vi "TEST - Wait Until Next ms Multiple.vi"(8 "error in (no error)":errorcluster) -> (0 "error out":errorcluster, 2 "pass":bool)   [LabVIEW 2020]
uses:
  source/library/openg_time.lvlib
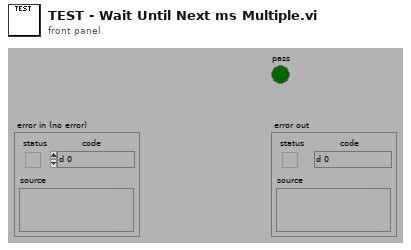
[diagram p1: front panel]
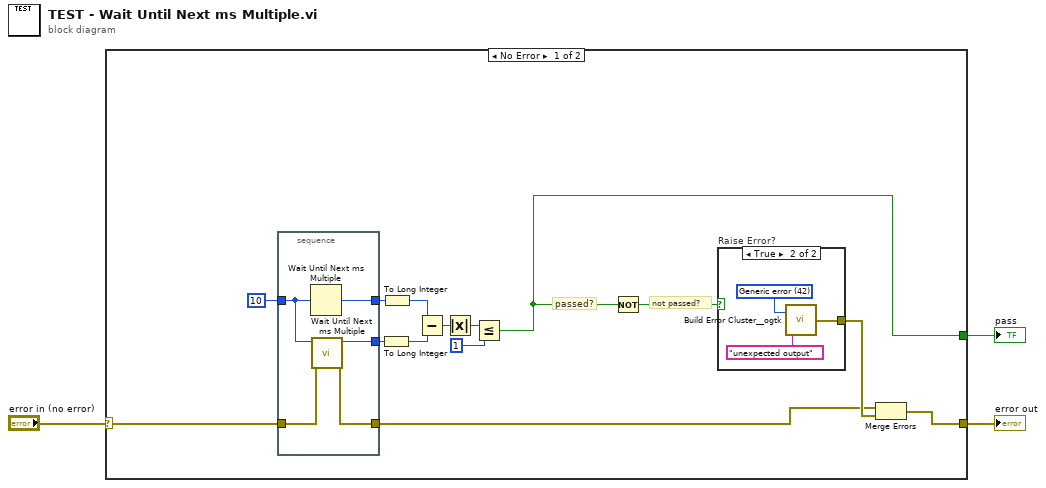
[diagram p0: block diagram]
diagram:
  n1 = case shown="No Error" "error in (no error)" {
    selector: "error in (no error)" -> [w13 w26]
    tunnel: [w11 _] -> w3
    tunnel: [w17 w26] -> w1
    frame No Error {
      # "not passed?"
      # "passed?"
      n2 = stacked-sequence {
        tunnel: [w21] -> w14
        tunnel: w13 -> [w22]
        tunnel: [w19] -> w8
        tunnel: u32 10 ("milliseconds to wait") -> [w20]
        tunnel: [w18] -> w9
        frame #0 {
          n3 = Wait Until Next ms Multiple(millisecond multiple=w20) -> (millisecond timer value=w18:u32)
          n4 = call "Wait Until Next ms Multiple.vi"("error in (no error)"=w22, "milliseconds to wait"=w20) -> ("error out"=w21:errorcluster, "millisecond timer value"=w19:u32)  [unwired: 8 in]
        }
      }
      n5 = To Long Integer(number=w8) -> (32bit integer=w5:i32)
      n6 = To Long Integer(number=w9) -> (32bit integer=w6:i32)
      n7 = Subtract(x=w6, y=w5) -> (x-y=w12:i32)
      n8 = Absolute Value(x=w12) -> (abs(x)=w7:i32)
      n9 = Less Or Equal?(x=w7, y=1) -> (x <= y?=w11:bool)
      n10 = Not(x=w11) -> (.not. x?=w15:bool)
      n11 = case "Raise Error?" shown="True" w15 {
        tunnel: [_ w23] -> w16
        frame False {
        }
        frame True {
          w24 = 42 items=["No error", "Argument error", "Memory is full", "Out of zone", "End of file", "File already open", "Generic file I/O error", "File not found", "File permission error", "Disk is full", "Duplicate path", "Too many files open", "System feature not enabled", "Resource file not found", "Cannot add resource", "Resource not found", "Image not found", "Image memory error", "Pen does not exist", "Config type invalid", "Config token not found", "Config parse error", "Config memory error", "Bad external code format", "Bad external code offset", "External code not present", "Null window", "Destroy window error", "Null menu", "Print aborted", "Bad print record", "Print driver error", "Windows error during printing", "Memory error during printing", "Print dialog error", "Generic print error", "Invalid device refnum", "Device not found", "Device parameter error", "Device unit error", "Cannot open device", "Device call aborted", "Generic error", "Cancelled by user", "Object ID too low", "Object ID too high", "Object not in heap", "Unknown heap", "Unknown object (invalid DefProc)", "Unknown object (DefProc not in table)", "Message out of range", "Invalid (null) method", "Unknown message", "Manager call not supported", "Bad address", "Network operation in progress", "Network operation timed out", "Connection is busy", "Network attribute not supported", "Network error", "Address in use", "System out of memory", "Connection aborted", "Connection refused", "Not connected", "Already connected", "Connection closed", "Initialization error (interapplication manager)", "Bad occurrence", "Wait on unbound occurrence handler", "Occurrence queue overflow", "Datalog type conflict", "Unused", "Unrecognized type (interapplication manager)", "Memory corrupt", "Failed to make temporary DLL", "Old CIN version", "Drag socket not found", "Failed to load drop-object", "Failed to register OLE object", "Failed to release OLE object", "Format specifier type mismatch", "Unknown format specifier", "Too few format specifiers", "Too many format specifiers", "Scan failed", "Newer CIN version", "Error converting to variant", "Runtime menu error", "Password tampered", "Variant attribute not found", "Incompatible variant data type", "Event data is not available", "Event Store is not present", "Occurrence is not found", "Event Queue is not created", "Event info is not available", "Refnum passed is NULL", "Error retrieving Class GUID", "Error retrieving CoClass GUID", "Error retrieving TypeLib GUID.", "Bad built application magic bytes.", "Specific driver is different from the specific driver associated with the Logical Name.", "There is no session opened to the class driver.", "Max Error", "MAX - Error with config objects", "MAX - Error loading configuration", "MAX - Group not supported"]
          n12 = call <userlib>:"Build Error Cluster__ogtk.vi"("String to Prepend to source (\"\")"="unexpected output" ("String to Prepend to source (\"\")"), "code"=w24) -> ("error out"=w23:errorcluster)
        }
      }
      n13 = Merge Errors(w14, w16) -> (w17:errorcluster)
    }
    frame Error {
    }
  }
  "pass" <- w3
  "error out" <- w1
